vi "To Variant.vi"(0 "Obj in":refnum<class "Noise.lvclass">, 11 "error in (no error)":errorcluster) -> (4 "Obj out":refnum<class "Noise.lvclass">, 8 "Array":variant[](array[variant]), 15 "error out":errorcluster)   [LabVIEW 2020, in "Noise.lvclass"]
uses:
  Noise.lvclass
  Noise.lvclass/Noise.ctl
  Waveform/Waveform.lvclass
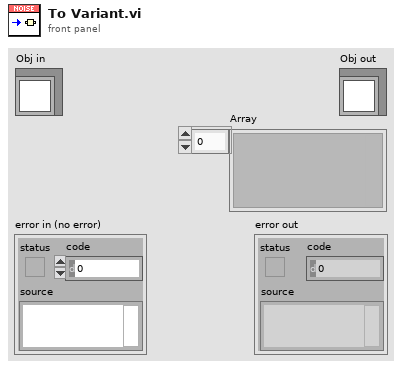
[diagram p1: front panel]
types:
  T1 = typedef "Noise.lvclass/Serialized.ctl" = cluster{"Seed":i32, "Tokens":i32, "InvFilt":bool, "Aweight":bool, "Weights":T2}
  T2 = typedef "Noise.lvclass/Weighting.ctl" = enum16{"White", "Pink"}
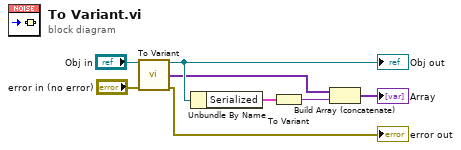
[diagram p0: block diagram]
diagram:
  n1 = call-parent "To Variant.vi"("Obj in"="Obj in", "error in (no error)"="error in (no error)") -> ("Obj out"=w3:refnum<class "Noise.lvclass">, "Array"=w2:variant[], "error out"=→"error out":errorcluster)  [unwired: 11 in]
  "Obj out" <- w3
  n2 = Unbundle By Name(w3) -> ("Serialized"=w4:T1)
  n3 = To Variant(anything=w4) -> (Variant=w5:variant)
  n4 = Build Array (concatenate)(w2, w5) -> (→"Array":variant[])
